vi "Close.vi"(7 "ignore already closed? (true)":bool=TRUE, 8 "error in (no error)":errorcluster, 11 "Subscription in":refnum<class "Subscription.lvclass">) -> (0 "error out":errorcluster)   [LabVIEW 2020, in "PV Access.lvlib" / "PVA Client.lvlib" / "Subscription.lvclass"]
doc: "Close the subscription."
uses:
  Subscription.lvclass
  PV Access.lvlib
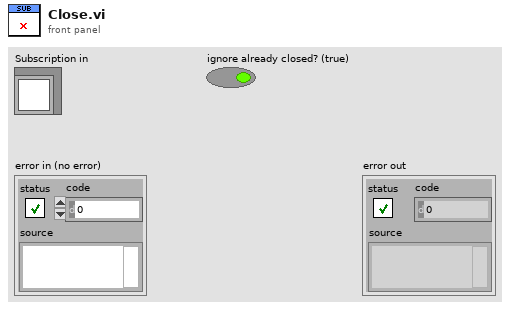
[diagram p1: front panel]
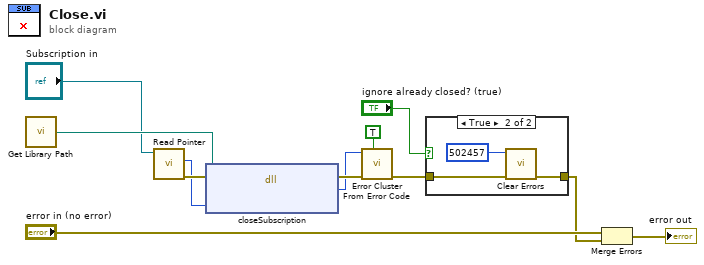
[diagram p0: block diagram]
diagram:
  n1 = call "Get Library Path.vi"() -> ("Path"=w12:path)  [unwired: 1 in]
  n2 = call-dynamic "Read Pointer.vi"("Pointer Base in"="Subscription in") -> ("error out"=w8:errorcluster, "Pointer"=w7:i64)  [unwired: 8 in, 1 out]
  n3 = dll-call lib="?" fn="closeSubscription"(path in=w12, error in=w8, "subscription"=w7) -> (error out=w10:errorcluster, "ret_code"=w9:i32)  [unwired: 2 in, 1 out]
  n4 = call <vilib>:"Error Cluster From Error Code.vi"("show call chain? (False)"=TRUE, "error in (no error)"=w10, "error code (0)"=w9) -> ("error out"=w3:errorcluster)  [unwired: 6 in]
  n5 = case shown="True" "ignore already closed? (true)" {
    tunnel: [w13 w15] -> w1
    tunnel: w3 -> [w13 w16]
    frame False {
    }
    frame True {
      n6 = call <vilib>:"Clear Errors.vi"("error in (no error)"=w16, "specific error code to clear (0: all)"=502457) -> ("error out"=w15:errorcluster)  [unwired: 4 in, 1 out]
    }
  }
  n7 = Merge Errors("error in (no error)", w1) -> (→"error out":errorcluster)
